vi "Configure Active Apparent Power.vi"(0 "VISA resource name":refnum<visa-resource-name>, 5 "Active Apparent Power Low Limit (0 VA)":dbl min=0.0 max=6000.0 format="%.1f", 7 "Active Apparent Power High Limit (0 VA)":dbl min=0.0 max=6000.0 format="%.1f", 11 "error in (no error)":errorcluster) -> (4 "VISA resource name out":refnum<visa-resource-name>, 15 "error out":errorcluster)   [LabVIEW 2016, in "APT 300XAC Series.lvlib"]
doc: "Configures the <B>Apparent Power Limits</B> of the power source instrument used for testing.\n\n<B>Range</B> : \n310XAC=0.0-1000\n320XAC=0.0-2000\n340XAC=0-4000\n360XAC=0-6000\n\n\nNote : Not supported in Program mode.\n\nThe Apparent Power Low-Limit defines the lower Apparent power limit of the output signal power APT300xAC Series Power Source can reach. Not reaching this value will fail the test\n\nThe Apparent Power High-Limit defines the higher Power limit of the output signal Power APT300xAC Series Power Source can reach. Crossing this value will fail the test"
uses:
  APT 300XAC Series.lvlib
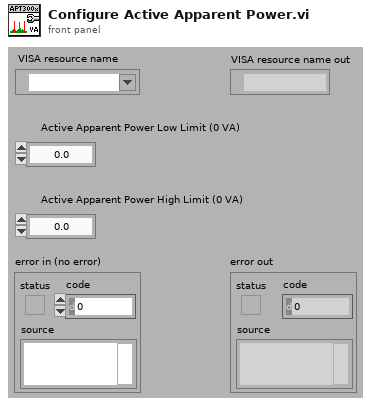
[diagram p1: front panel]
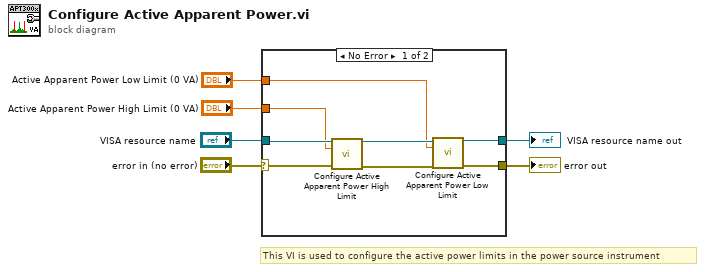
[diagram p0: block diagram]
diagram:
  # "This VI is used to configure the active power limits in the power source instrument"
  n1 = case shown="No Error" "error in (no error)" {
    selector: "error in (no error)" -> [w14 w15]
    tunnel: "VISA resource name" -> [w13 w16]
    tunnel: [w9 w16] -> w5
    tunnel: [w8 w15] -> w4
    tunnel: "Active Apparent Power High Limit (0 VA)" -> [w12 _]
    tunnel: "Active Apparent Power Low Limit (0 VA)" -> [w7 _]
    frame No Error {
      n2 = call "Configure Active Apparent Power High Limit.vi"("VISA resource name"=w13, "Active Apparent Power (1000 Hz)"=w12, "error in (no error)"=w14) -> ("VISA resource name out"=w11:refnum<visa-resource-name>, "error out"=w10:errorcluster)  [unwired: 11 in]
      n3 = call "Configure Active Apparent Power Low Limit.vi"("VISA resource name"=w11, "Apparent Power Low Limit (40.0)"=w7, "error in (no error)"=w10) -> ("VISA resource name out"=w9:refnum<visa-resource-name>, "error out"=w8:errorcluster)  [unwired: 11 in]
    }
    frame Error {
    }
  }
  "error out" <- w4
  "VISA resource name out" <- w5
